vi "Main Body.vi"(8 "error in (no error)":errorcluster, 10 "File Actor In":refnum<class "File Actor.lvclass">, 11 "Exe Write Main CMD in":refnum<class "Exe Write Main CMD.lvclass">) -> (0 "error out":errorcluster)   [LabVIEW 2016, in "Controller.lvlib" / "Exe Write Main CMD.lvclass"]
uses:
  Exe Write Main CMD.lvclass
  File Actor/File Actor.lvclass
  Exe Write Main CMD.lvclass/Exe Write Main CMD.ctl
  File Actor/File Actor.lvclass/File Actor.ctl
  <vilib>/MSR Consulting, LLC/General Reuse/Data/Data.lvclass
  File Actor/Read Save DVR.vi
  File Actor/Read File DVR.vi
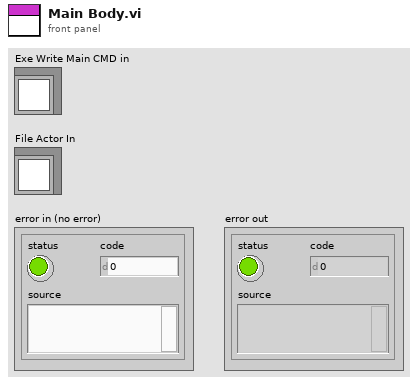
[diagram p1: front panel]
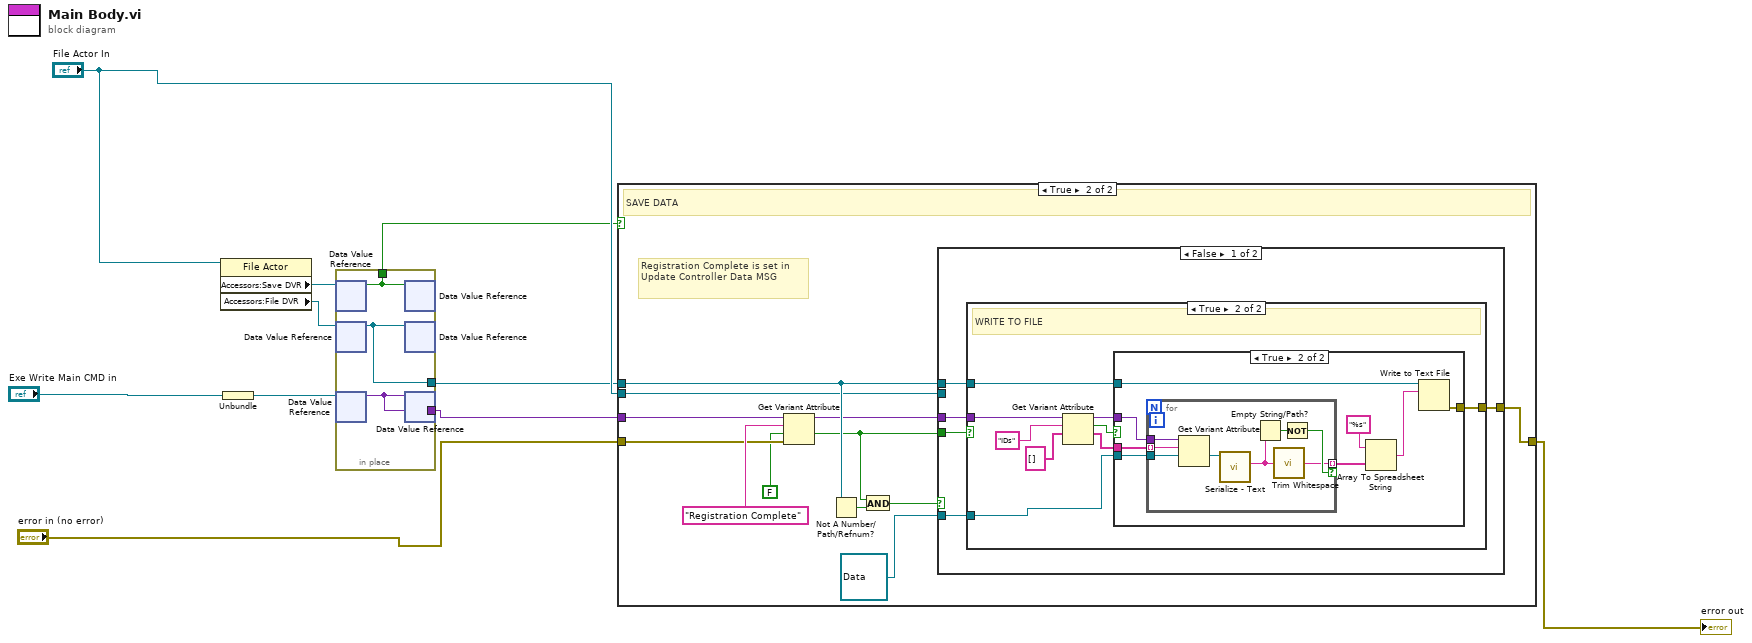
[diagram p0: block diagram]
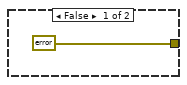
[diagram p4: hidden frame]
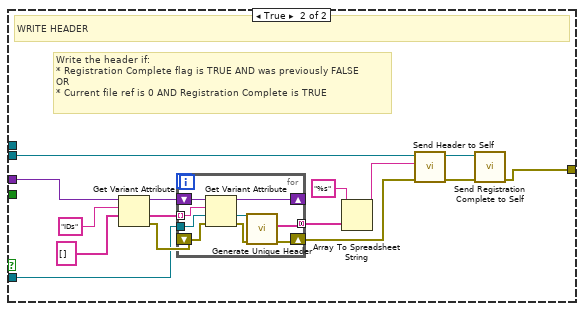
[diagram p5: hidden frame]
diagram:
  n1 = property class="File Actor"(reference="File Actor In") -> ("Accessors:Save DVR"=w1:refnum<data-value>, "Accessors:File DVR"=w2:refnum<data-value>)  [unwired: 1 in, 2 out]
  n2 = Unbundle("Exe Write Main CMD in") -> (w6:refnum<data-value>)
  n3 = in-place {
    in-place-border: [w13] -> w4
    in-place-border: [w12] -> w5
    in-place-border: [w11] -> w7
    n4 = in-place-dvr #1(w1) -> (w12:bool)  [unwired: 1 out]
    n5 = in-place-dvr #2(w2) -> (w13:refnum<file>)  [unwired: 1 out]
    n6 = in-place-dvr #3(w6) -> (w11:variant)  [unwired: 1 out]
    n7 = in-place-dvr #1(w12) -> ()  [unwired: 2 out]
    n8 = in-place-dvr #2(w13) -> ()  [unwired: 2 out]
    n9 = in-place-dvr #3(w11) -> ()  [unwired: 2 out]
  }
  n10 = case shown="True" w5 {
    tunnel: [w14 w26] -> w10
    tunnel: w4 -> [_ w23]
    tunnel: "error in (no error)" -> [w14 w20]
    tunnel: w7 -> [_ w25]
    tunnel: "File Actor In" -> [_ w19]
    frame False {
      # "NO SAVE"
    }
    frame True {
      # "Registration Complete is set in Update Controller Data MSG"
      # "SAVE DATA"
      n11 = Get Variant Attribute(Variant=w25, name="Registration Complete", default value (empty Variant)=FALSE, error in=w20) -> (duplicate Variant=w18:variant, value=w21:bool)  [unwired: 2 out]
      n12 = Not A Number/Path/Refnum?(number/path/refnum=w23) -> (NaN/Path/Refnum?=w22:bool)
      n13 = And(x=w21, y=w22) -> (x .and. y?=w16:bool)
      n14 = case shown="False" w16 {
        tunnel: [w31 w58] -> w26
        tunnel: w23 -> [w30 _]
        tunnel: w18 -> [w29 w72]
        tunnel: w21 -> [w28 _]
        tunnel: w19 -> [_ w63]
        tunnel: refnum<class "Data.lvclass"> refnum ("Base Data Lib:Data") -> [w27 w64]
        frame False {
          n15 = case shown="True" w28 {
            tunnel: [_ w40] -> w31
            tunnel: w30 -> [_ w38]
            tunnel: w29 -> [_ w39]
            tunnel: w27 -> [_ w32]
            frame False {
            }
            frame True {
              # "WRITE TO FILE"
              n16 = Get Variant Attribute(Variant=w39, name="IDs", default value (empty Variant)=string[] []) -> (duplicate Variant=w33:variant, found=w34:bool, value=w35:string[])  [unwired: 1 in, 1 out]
              n17 = case shown="True" w34 {
                tunnel: w35 -> [_ w49]
                tunnel: w33 -> [_ w48]
                tunnel: w32 -> [_ w47]
                tunnel: w38 -> [_ w44]
                tunnel: [errorcluster {"status"=FALSE, "code"=0, "source"=""} ("error out") w43] -> w40
                frame False {
                }
                frame True {
                  n18 = for {
                    tunnel: w49 -> [w52] mode=indexing
                    tunnel: w48 -> [w57]
                    tunnel: w47 -> [w56]
                    tunnel: [w53] -> w46 mode=indexing if=w54
                    n19 = Get Variant Attribute(Variant=w57, name=w52, default value (empty Variant)=w56) -> (value=w51:refnum<class "Data.lvclass">)  [unwired: 1 in, 3 out]
                    n20 = call-dynamic "Serialize - Text.vi"("Data in"=w51) -> ("Serialized Text"=w50:string)  [unwired: 8 in, 2 out]
                    n21 = Empty String/Path?(string/path=w50) -> (empty?=w55:bool)
                    n22 = call <vilib>:"Trim Whitespace.vi"("string"=w50) -> ("trimmed string"=w53:string)  [unwired: 1 in]
                    n23 = Not(x=w55) -> (.not. x?=w54:bool)
                  }
                  n24 = Array To Spreadsheet String(array=w46, 3:"%s" ("format string")) -> (spreadsheet string=w42:string)  [unwired: 1 in]
                  n25 = Write to Text File(file (use dialog)=w44, text=w42) -> (error out=w43:errorcluster)  [unwired: 2 in, 2 out]
                }
              }
            }
          }
        }
        frame True {
          # "Write the header if:\n* Registration Complete flag is TRUE AND was previously FALSE\nOR \n* Current file ref is 0 AND Registration Complete is TRUE"
          # "WRITE HEADER"
          n26 = Get Variant Attribute(Variant=w72, name="IDs", default value (empty Variant)=string[] []) -> (duplicate Variant=w68:variant, value=w69:string[], error out=w65:errorcluster)  [unwired: 1 in, 1 out]
          n27 = for {
            tunnel: w69 -> [w81] mode=indexing
            tunnel: w64 -> [w79]
            tunnel: [w75] -> w67 mode=concatenating
            shift-right: [w73] -> w62
            shift-left: w65 -> [w78]
            shift-right: [w77] -> _
            shift-left: w68 -> [w80]
            n28 = Get Variant Attribute(Variant=w80, name=w81, default value (empty Variant)=w79, error in=w78) -> (duplicate Variant=w77:variant, value=w76:refnum<class "Data.lvclass">, error out=w74:errorcluster)  [unwired: 1 out]
            n29 = call-dynamic "Generate Unique Header.vi"("error in"=w74, "Data in"=w76) -> ("error out"=w73:errorcluster, "Header"=w75:string[])  [unwired: 7 in, 1 out]
          }
          n30 = Array To Spreadsheet String(array=w67, 3:"%s" ("format string")) -> (spreadsheet string=w61:string)  [unwired: 1 in]
          n31 = call "Send Header to Self.vi"("error in"=w62, "Header"=w61, "File Actor in"=w63) -> ("error out"=w59:errorcluster, "File Actor out"=w60:refnum<class "File Actor.lvclass">)  [unwired: 7 in]
          n32 = call "Send Registration Complete to Self.vi"("error in (no error)"=w59, "File Actor in"=w60) -> ("error out"=w58:errorcluster)  [unwired: 8 in, 1 out]
        }
      }
    }
  }
  "error out" <- w10
